vi "Ensure Default Fills.vi"(8 "error in":errorcluster, 11 "SpreadsheetDoc in":refnum<k24>) -> (0 "error out":errorcluster, 3 "SpreadsheetDoc out":refnum<k24>)   [LabVIEW 2021, in "Open Xml.lvlib"]
uses:
  Open Xml.lvlib
  D:/git/Open-Xml-LabVIEW/dll/DocumentFormat.OpenXml.dll
  dll/DocumentFormat.OpenXml.dll
  D:/git/Open-Xml-LabVIEW/dll/DocumentFormat.OpenXml.Framework.dll
  dll/DocumentFormat.OpenXml.Framework.dll
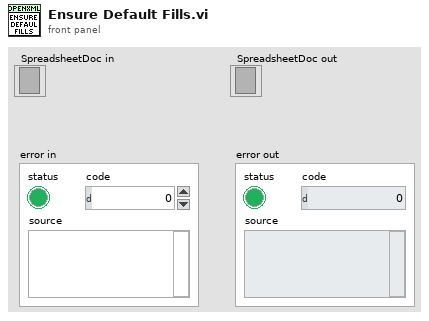
[diagram p1: front panel]
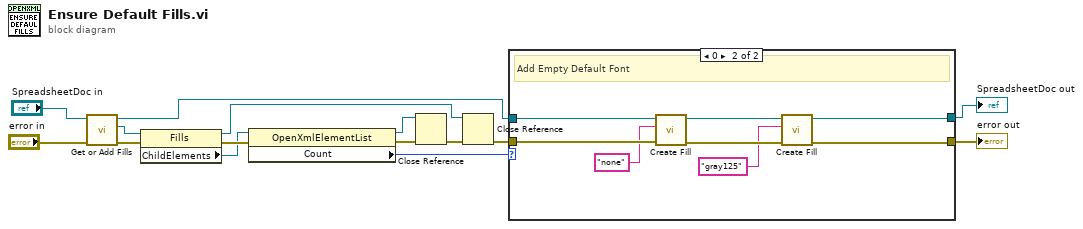
[diagram p0: block diagram]
diagram:
  n1 = call "Get or Add Fills.vi"("error in"="error in", "SpreadsheetDoc in"="SpreadsheetDoc in") -> ("error out"=w11:errorcluster, "Fills"=w10:refnum<k24>, "SpreadsheetDoc out"=w7:refnum<k24>)  [unwired: 7 in]
  n2 = property class="Fills"(reference=w10, error in=w11) -> (reference out=w2:refnum<k24>, error out=w9:errorcluster, "ChildElements"=w4:refnum<k24>)
  n3 = property class="OpenXmlElementList"(reference=w4, error in=w9) -> (reference out=w1:refnum<k24>, error out=w6:errorcluster, "Count"=w8:i32)
  n4 = Close Reference(reference=w1, error in (no error)=w6) -> (error out=w5:errorcluster)
  n5 = Close Reference(reference=w2, error in (no error)=w5) -> (error out=w3:errorcluster)
  n6 = case shown="0" w8 {
    tunnel: w7 -> [w16 w25]
    tunnel: w3 -> [w17 w24]
    tunnel: [w17 w21] -> w14
    tunnel: [w16 w19] -> w15
    frame Default {
      # "Default"
    }
    frame 0 {
      # "Add Empty Default Font"
      n7 = call "Create Fill.vi"("error in"=w24, "PatternType"="none" ("value"), "SpreadsheetDoc in"=w25) -> ("error out"=w22:errorcluster, "SpreadsheetDoc out"=w20:refnum<k24>)  [unwired: 7 in]
      n8 = call "Create Fill.vi"("error in"=w22, "PatternType"="gray125", "SpreadsheetDoc in"=w20) -> ("error out"=w21:errorcluster, "SpreadsheetDoc out"=w19:refnum<k24>)  [unwired: 7 in]
    }
  }
  "SpreadsheetDoc out" <- w15
  "error out" <- w14
